vi "Initialize.vi"(8 "error in":errorcluster, 9 "PPLs Folder Path":path, 10 "INI File Path":path, 11 "Device":string) -> (0 "error out":errorcluster, 3 "EXFO out":refnum<class "EXFO.lvclass">)   [LabVIEW 2018, in "EXFO.lvlib" / "EXFO.lvclass"]
doc: "Initialize routine - Loads class specifier and Resource ID from the configuration file. This allows for all coding to use the parent method and implementation in TestStand as a packed project library. \n\nThere is no child class override for this function call. *DO NOT MODIFY*\n\nAuthor: Ron Dexter\nCompany: Luminar\nModified: 5/20/2018"
uses:
  EXFO.lvclass
  EXFO.lvclass/EXFO.ctl
  PPLs/Configuration/Configuration.lvlibp/Configuration.lvclass
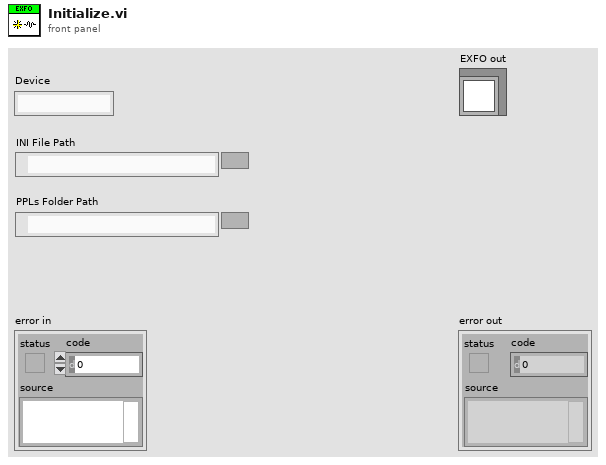
[diagram p1: front panel]
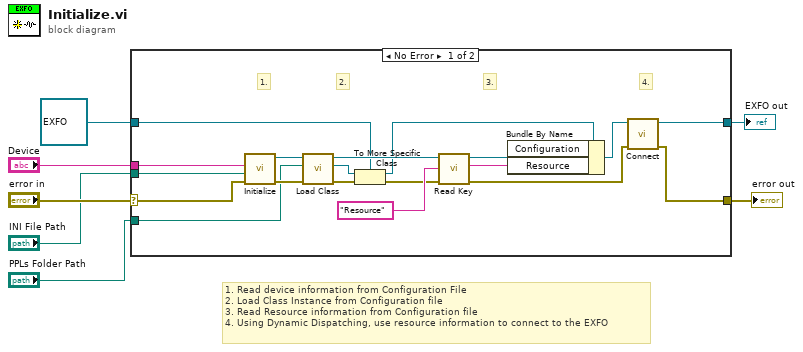
[diagram p0: block diagram]
diagram:
  # "1. Read device information from Configuration File\n2. Load Class Instance from Configuration file\n3. Read Resource information from Configuration file\n4. Using Dynamic Dispatching, use resource information to connect to the EXFO"
  n1 = case shown="No Error" "error in" {
    selector: "error in" -> [w26 w28]
    tunnel: [w19 w28] -> w6
    tunnel: [w21 w27] -> w4
    tunnel: refnum<class "EXFO.lvclass"> refnum ("EXFO in") -> [w12 w27]
    tunnel: "Device" -> [w25 _]
    tunnel: "INI File Path" -> [w9 _]
    tunnel: "PPLs Folder Path" -> [w8 _]
    frame No Error {
      # "4."
      # "3."
      # "2."
      # "1."
      n2 = call "Initialize.vi"("error in"=w26, "INI File Path"=w9, "Device"=w25) -> ("error out"=w16:errorcluster, "Configuration out"=w18:refnum<class "Configuration.lvclass">)  [unwired: 7 in]
      n3 = call "Load Class.vi"("error in"=w16, "PPLs Folder Path"=w8, "Configuration in"=w18) -> ("error out"=w15:errorcluster, "Class out"=w13:refnum<class>, "Configuration out"=w17:refnum<class "Configuration.lvclass">)  [unwired: 6 in]
      n4 = To More Specific Class(target class=w12, reference=w13, error in=w15) -> (specific class reference=w11:refnum<class "EXFO.lvclass">, error out=w14:errorcluster)
      n5 = call "Read Key.vi"("Key:"="Resource" ("Search Value"), "error in"=w14, "Configuration in"=w17) -> ("error out"=w20:errorcluster, "Value"=w23:string, "Configuration out"=w10:refnum<class "Configuration.lvclass">)  [unwired: 6 in]
      n6 = Bundle By Name(cluster=w11, "Configuration"=w10, "Resource"=w23) -> (w22:refnum<class "EXFO.lvclass">)
      n7 = call-dynamic "Connect.vi"("error in (no error)"=w20, "EXFO in"=w22) -> ("error out"=w19:errorcluster, "EXFO out"=w21:refnum<class "EXFO.lvclass">)  [unwired: 8 in]
    }
    frame Error {
    }
  }
  "error out" <- w6
  "EXFO out" <- w4
